vi "parse parameter IDs and Values list.vi"(11 "Arg":string) -> (3 "Array":dbl[][](array[numeric]))   [LabVIEW 2020, in "SITK.lvclass"]
uses:
  SITK.lvclass
panel:
  out "array":string[](array[string])
  # "example input\n2:3,4:5\nI.e. par id 2, value 3"
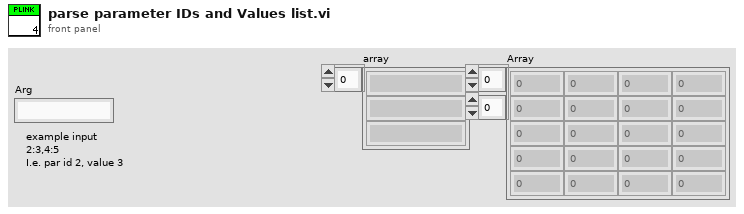
[diagram p1: front panel]
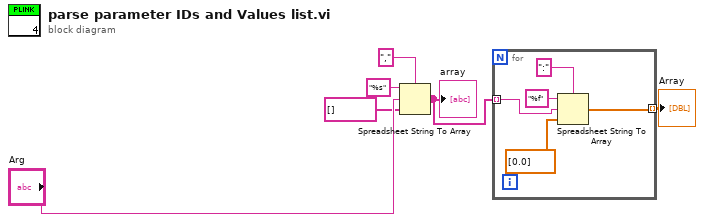
[diagram p0: block diagram]
diagram:
  n1 = Spreadsheet String To Array(delimiter (Tab)=",", format string="%s", spreadsheet string="Arg", array type (2D Dbl)=string[] []) -> (array=w2:string[])
  "array" <- w2
  n2 = for {
    tunnel: w2 -> [w9] mode=indexing
    tunnel: [w8] -> w1 mode=indexing
    n3 = Spreadsheet String To Array(delimiter (Tab)=":", format string="%f", spreadsheet string=w9, array type (2D Dbl)=dbl[] [0.0]) -> (array=w8:dbl[])
  }
  "Array" <- w1
